vi "Exp no 7a Application Using WHILE LOOP.vi"() -> ()   [LabVIEW 2010]
panel:
  out "Sum of N Odd Numbers":dbl
  in  "N":dbl
  # "SUM OF N ODD NUMBERS"
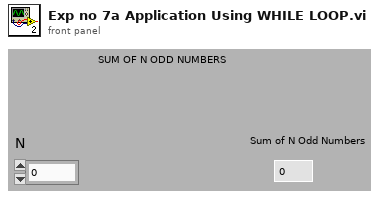
[diagram p1: front panel]
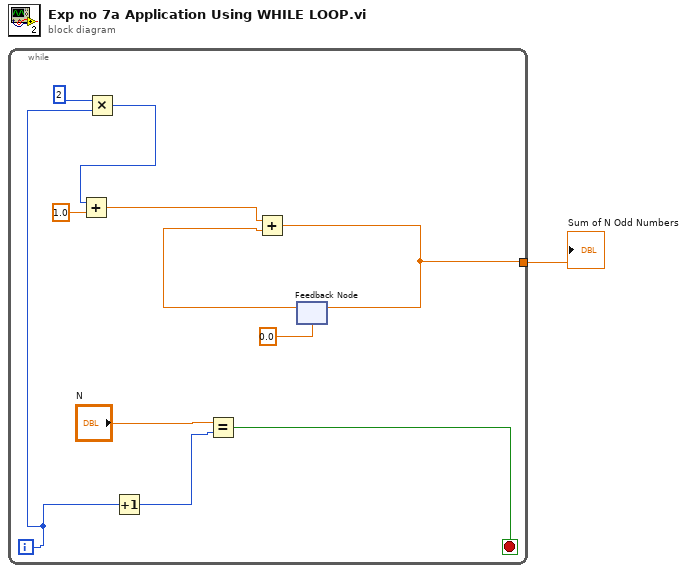
[diagram p0: block diagram]
diagram:
  n1 = while {
    tunnel: [w2] -> w1
    i -> [w7]
    stop <- w10 stop-if-true
    n2 = Multiply(x=2 ("y"), y=w7) -> (x*y=w8:i32)
    n3 = Add(x=w8, y=1.0) -> (x+y=w3:dbl)
    n4 = Increment(x=w7) -> (x+1=w11:i32)
    n5 = Equal?(x="N", y=w11) -> (x = y?=w10:bool)
    n6 = feedback #1(0.0) -> (w5:dbl)
    n7 = Add(x=w3, y=w5) -> (x+y=w2:dbl)
    n8 = feedback-in #1(w2) -> ()
  }
  "Sum of N Odd Numbers" <- w1
